vi "LVClass_CorrectionDataManager GetDiagnosticsSingularVector.vi"(0 "CorrectionDataManager in":refnum<class "CorrectionDataManager.lvclass">, 11 "error in (no error)":errorcluster) -> (4 "CorrectionDataManager out":refnum<class "CorrectionDataManager.lvclass">, 6 "ArrayOfSingularValues":dbl[](array[numeric]), 15 "error out":errorcluster)   [LabVIEW 2020, in "CorrectionDataManager.lvclass"]
doc: "Get vector of singular values.\n\n<B>corrdata_managerIn</B> : CorrDataManager object.\n<B>corrdata_managerOut</B> : CorrDataManager object.\n<B>singular_vector</B> : Array of influences, sorted in descending order."
uses:
  CorrectionDataManager.lvclass
  CorrectionDataManager.lvclass/CorrectionDataManager.ctl
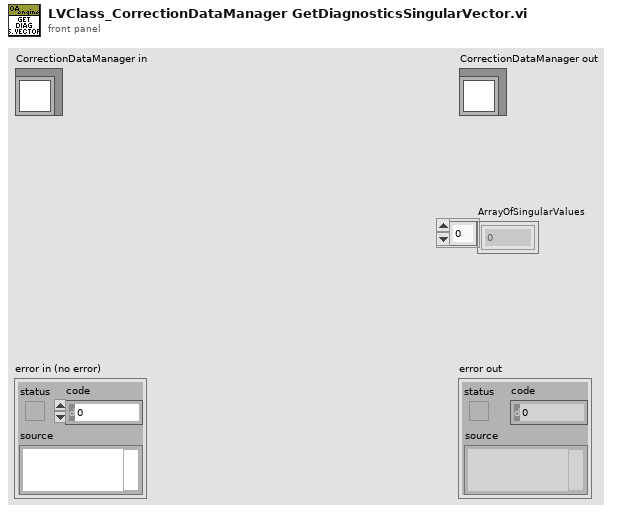
[diagram p1: front panel]
types:
  T1 = typedef "ClassID.ctl" = i64
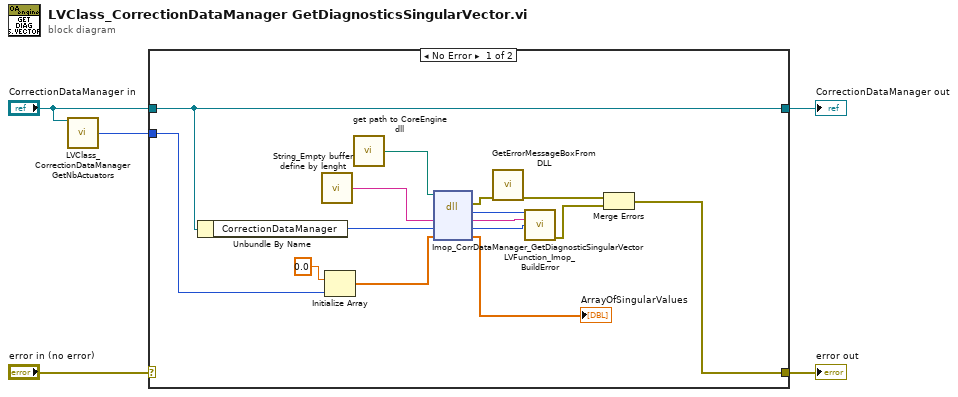
[diagram p0: block diagram]
diagram:
  n1 = call "LVClass_CorrectionDataManager GetNbActuators.vi"("CorrectionDataManager in"="CorrectionDataManager in") -> ("Nb actuators"=w1:i32)  [unwired: 12 in, 2 out]
  n2 = case shown="No Error" "error in (no error)" {
    selector: "error in (no error)" -> [_ w22]
    tunnel: [w12 w22] -> w4
    tunnel: [w13 w21] -> w5
    tunnel: "CorrectionDataManager in" -> [w13 w21]
    tunnel: w1 -> [w8 _]
    frame No Error {
      n3 = Unbundle By Name(w13) -> ("CorrectionDataManager"=w11:T1)
      n4 = call "String_Empty buffer define by lenght.vi"() -> ("Empty buffer"=w18:string)  [unwired: 1 in]
      n5 = Initialize Array(sgl 0.0, w8) -> (w7:sgl[])
      n6 = call "get path to CoreEngine dll.vi"() -> ("path to wavekit library"=w17:path)  [unwired: 14 in, 1 out]
      n7 = dll-call lib="D:/SOFTware/HASO_v3/SVN_trunk/ImOpCoreEngine4_LV2011/DLLs/c_interface_vc100.dll" fn="Imop_CorrDataManager_GetDiagnosticSingularVector"(path in=w17, "message"=w18, "WavefrontCorrection"=w11, "Singular_Vector"=w7) -> (error out=w16:errorcluster, "return type"=w20:i32, "message"=w19:string, "WavefrontCorrection"=w6:i64, "Singular_Vector"=→"ArrayOfSingularValues":sgl[])  [unwired: 2 in, 1 out]
      n8 = call "GetErrorMessageBoxFromDLL.vi"("error IN"=w16) -> ("error OUT"=w15:errorcluster)  [unwired: 10 in]
      n9 = call "LVFunction_Imop_BuildError.vi"("code"=w20, "String to Prepend to source (\"\")"=w19, "Adresse"=w6) -> ("error out"=w14:errorcluster)  [unwired: 12 in]
      n10 = Merge Errors(w15, w14) -> (w12:errorcluster)
    }
    frame Error {
    }
  }
  "error out" <- w4
  "CorrectionDataManager out" <- w5
